vi "Enum Queue State Machine.vi"   [LabVIEW 2020, in "Enum Queue State Machine.lvlib"]
uses:
  Enum Queue State Machine.lvlib
  Enum Queue/Enqueue Enum (single).vi
  Toolbox/Controls State (array).vi
  Enum Queue/Enqueue Enum (array).vi
types:
  T1 = enum16{"User Event", "Initialize Core Data", "Data: Initialize", "Data: Cleanup", "UI: Initialize", "UI: Set Cursor State", "UI: Controls State", "UI: Front Panel State", "Macro: Initialize", "Macro: Exit", "Error Handler", "Exit"}
  T2 = enum32{"Invalid", "Standard", "Closed", "Hidden", "Minimized", "Maximized"}
  T3 = enum32{"invalid app kind", "Development System", "Run Time System", "Student Edition", "Embedded LabVIEW", "Evaluation", "Custom"}
  T4 = cluster{refnum<vi>[], "Disabled":enum8{"Enabled", "Disabled", "Disabled and Grayed Out"}}
  T5 = cluster{"Core":cluster{"Current VI Reference":refnum<vi>, "Close Panel on Exit?":bool}, "Data":bool}
  T6 = cluster{"Current VI Reference":refnum<vi>, "Close Panel on Exit?":bool}
  T7 = enum8{"Enabled", "Disabled", "Disabled and Grayed Out"}
  T8 = enum16{"User Event", "Initialize Core Data", "Data: Initialize", "Data: Cleanup", "UI: Initialize", "UI: Set Cursor State", "UI: Controls State", "UI: Front Panel State", "Macro: Initialize", "Macro: Exit", "Error Handler", "Exit"}[]
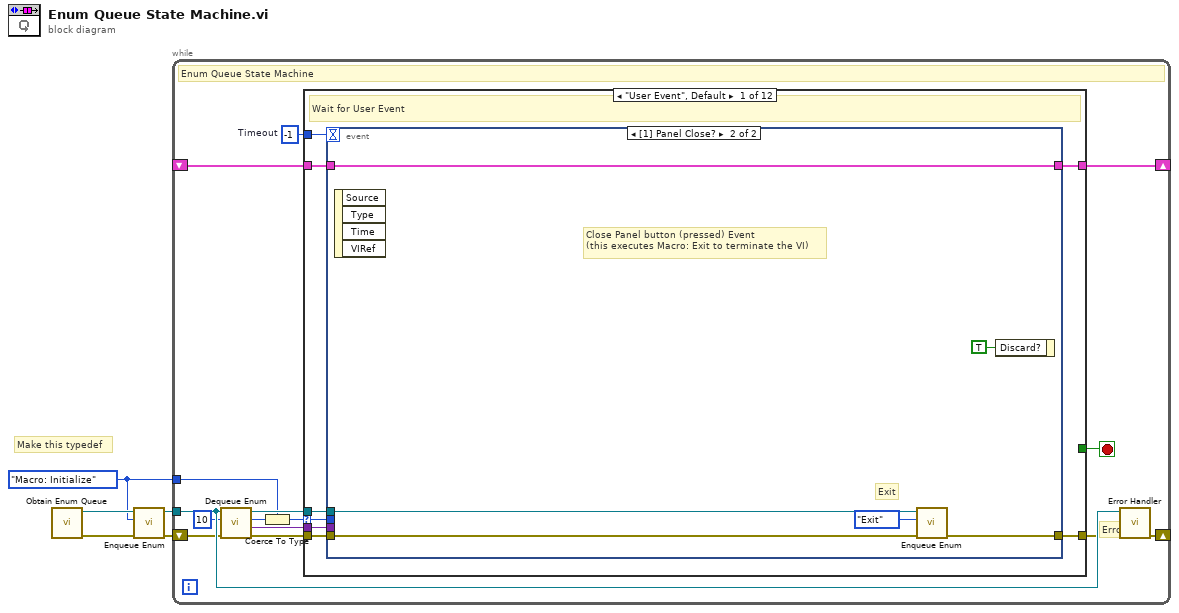
[diagram p0: block diagram]
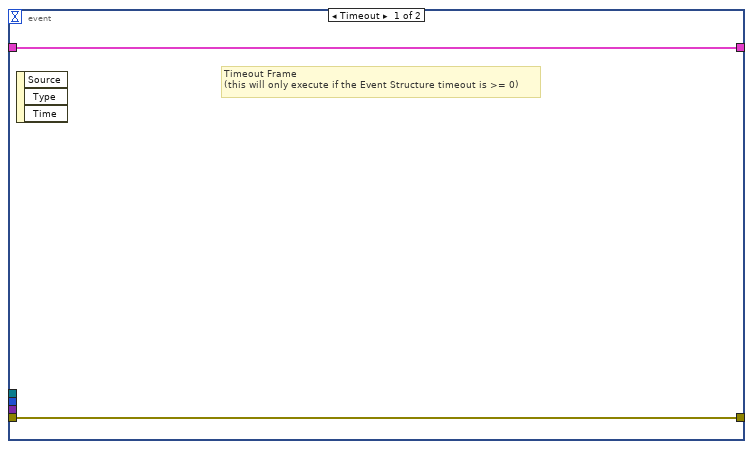
[diagram p2: hidden frame]
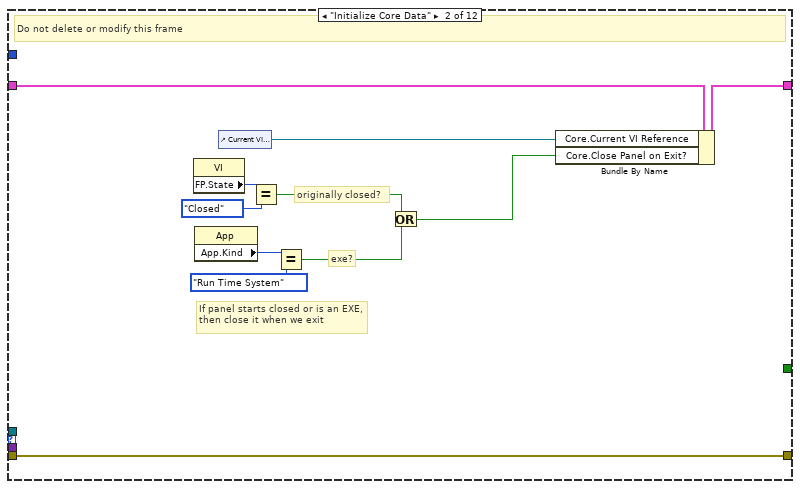
[diagram p3: hidden frame]
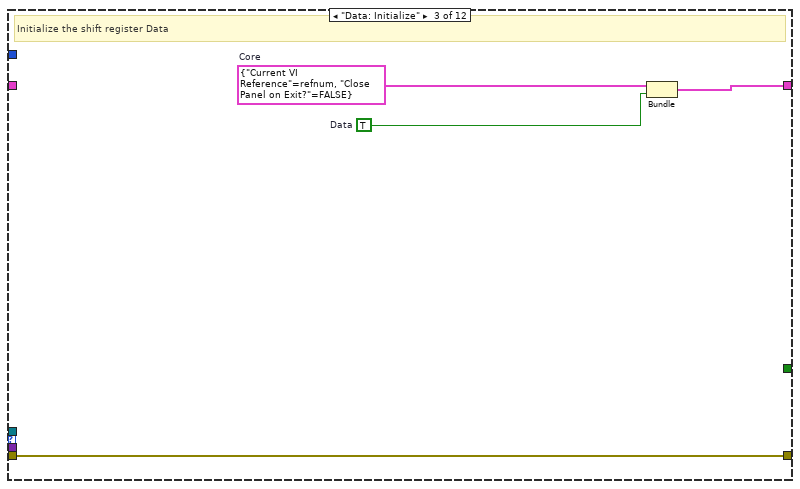
[diagram p4: hidden frame]
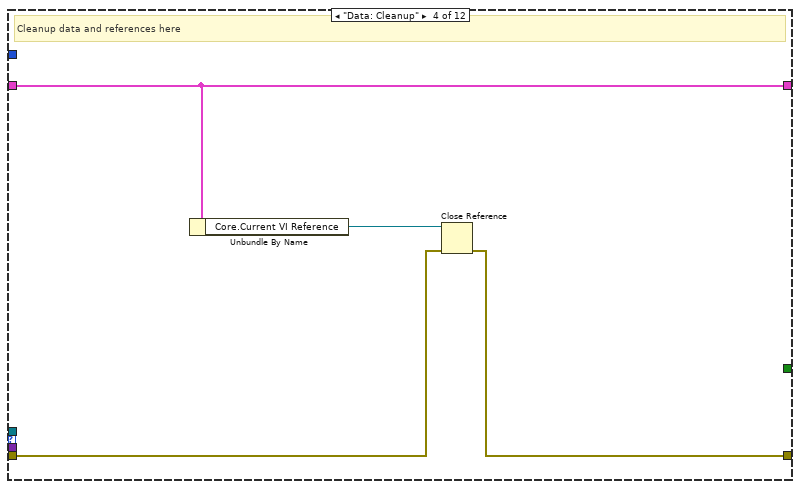
[diagram p5: hidden frame]
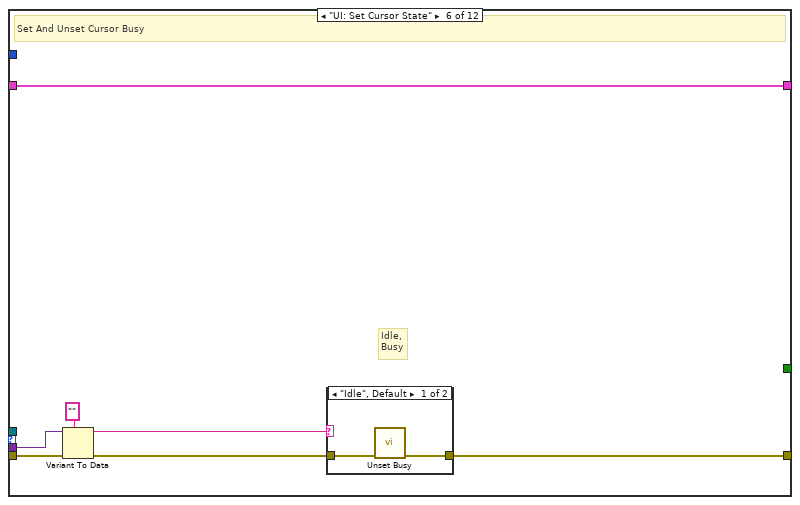
[diagram p7: hidden frame]
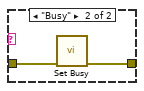
[diagram p8: hidden frame]
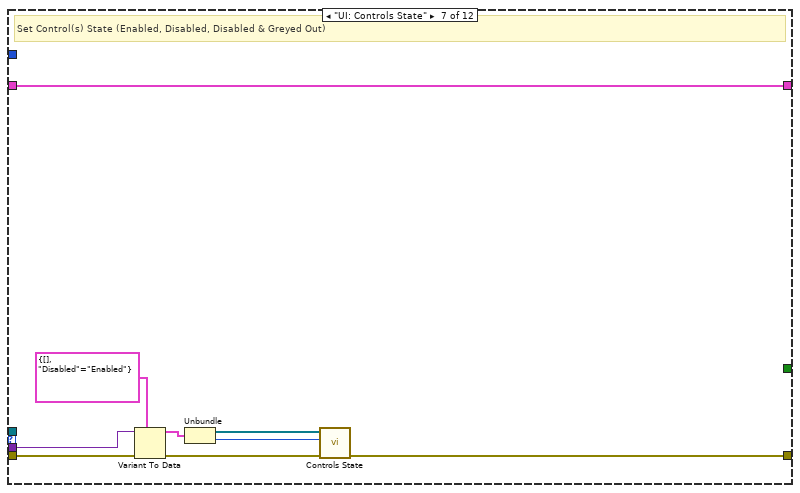
[diagram p9: hidden frame]
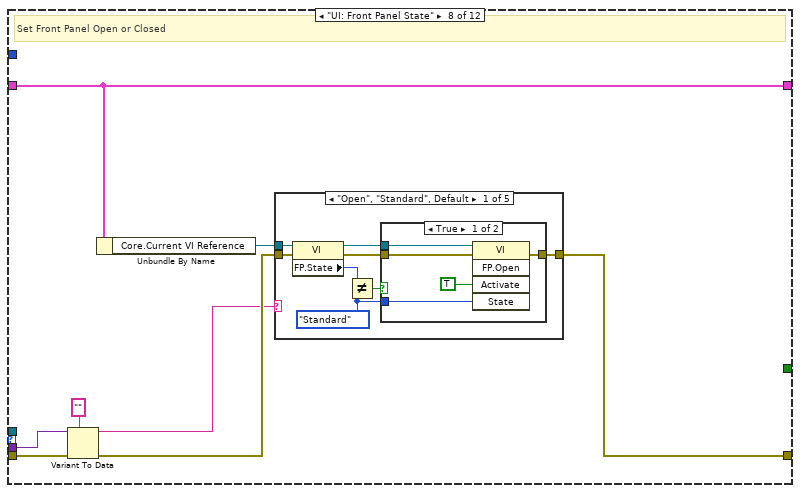
[diagram p10: hidden frame]
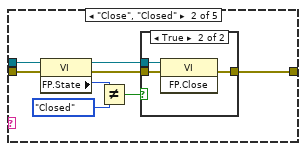
[diagram p12: hidden frame]
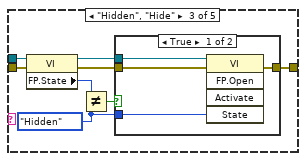
[diagram p14: hidden frame]
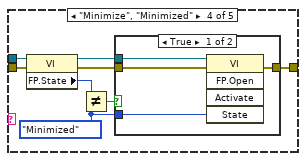
[diagram p16: hidden frame]
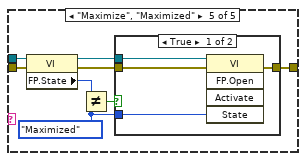
[diagram p18: hidden frame]
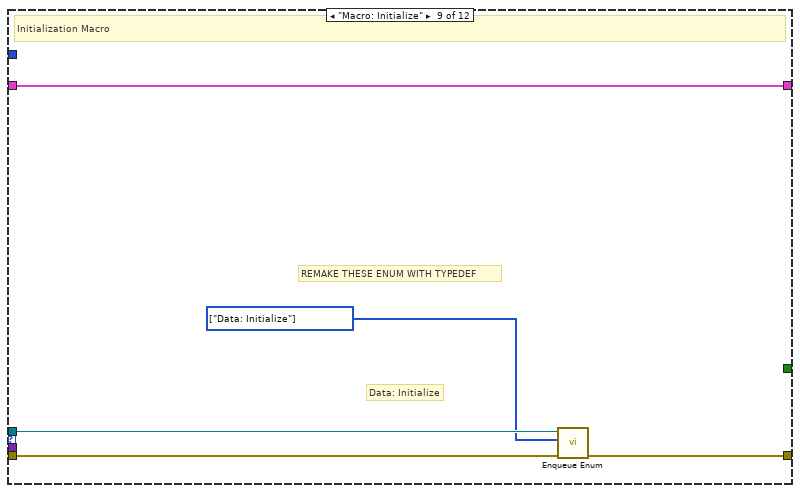
[diagram p20: hidden frame]
diagram:
  w1 = T1."Macro: Initialize"
  # "Make this typedef"
  n1 = call "Obtain Enum Queue.vi"() -> ("error out"=w2:errorcluster, "Queue Out"=w5:refnum<queue>)  [unwired: 10 in]
  n2 = call-poly "Enqueue Enum.vi"("error in"=w2, "State"=w1, "Queue In"=w5) -> ("error out"=w3:errorcluster, "Queue Out"=w4:refnum<queue>)  [unwired: 7 in]
  n3 = while {
    tunnel: w4 -> [w20]
    shift-right: [w6] -> _
    shift-left: w3 -> [w19]
    tunnel: w1 -> [w13]
    shift-right: [w11] -> _
    shift-left: _ -> [w12]
    stop <- w9 stop-if-true
    w10 = -1  # Timeout
    # "Error"
    # "Enum Queue State Machine"
    n4 = call "Dequeue Enum.vi"("error in"=w19, "Timeout ms (-1)"=10, "Queue In"=w20) -> ("error out"=w18:errorcluster, "Data"=w16:variant, "State"=w15:i32, "Queue Out"=w17:refnum<queue>)  [unwired: 5 in]
    n5 = Coerce To Type(0:w15, 1:w13) -> (2:w14:T1)
    n6 = case shown="\"User Event\", Default" w14 {
      selector: w14 -> [w21 _ _ _ _ _ _ _ _ _ _ _]
      tunnel: w18 -> [w28 w37 w51 w55 w57 w62 w76 w82 w154 w160 w175 w183]
      tunnel: w17 -> [w23 _ _ _ _ _ _ _ w152 w157 w174 w181]
      tunnel: w16 -> [w22 _ _ _ _ w60 w75 w80 _ _ _ _]
      tunnel: [w27 w37 w51 w54 w57 w63 w71 w84 w153 w163 w172 w182] -> w7
      tunnel: w12 -> [w25 w47 _ w53 w56 w64 w77 w83 w155 w161 w176 w185]
      tunnel: [w24 w46 w50 w53 w56 w64 w77 w83 w155 w161 w176 w185] -> w11
      tunnel: w10 -> [w26 _ _ _ _ _ _ _ _ _ _ _]
      tunnel: [_ _ _ _ _ _ _ _ _ _ _ TRUE] -> w9
      frame "User Event", Default {
        # "Wait for User Event"
        n7 = event shown="[1] Panel Close?" {
          selector: _ -> [_ _]
          dyn-events: _ -> [_ _]
          timeout: w26 -> [_ _]
          tunnel: w28 -> [w30 w34]
          tunnel: [w30 w33] -> w27
          tunnel: w25 -> [w29 w36]
          tunnel: [w29 w36] -> w24
          tunnel: w23 -> [_ w32]
          tunnel: w22 -> [_ _]
          tunnel: w21 -> [_ _]
          event Timeout {
            # "Timeout Frame\n(this will only execute if the Event Structure timeout is >= 0)"
            n8 = event-data() -> ()  [unwired: 1 in, 3 out]
          }
          event Panel Close? {
            # "Exit"
            # "Close Panel button (pressed) Event\n(this executes Macro: Exit to terminate the VI)"
            n9 = event-data() -> ()  [unwired: 1 in, 4 out]
            n10 = call-poly "Enqueue Enum.vi"("error in"=w34, "State"=T1."Exit", "Queue In"=w32) -> ("error out"=w33:errorcluster)  [unwired: 7 in, 1 out]
            n11 = event-data("Discard?"=TRUE) -> ()  [unwired: 1 in, 1 out]
          }
        }
      }
      frame "Initialize Core Data" {
        # "originally closed?"
        # "exe?"
        # "If panel starts closed or is an EXE, then close it when we exit"
        # "Do not delete or modify this frame"
        n12 = property class="VI"() -> ("FP.State"=w42:T2)  [unwired: 2 in, 2 out]
        n13 = property class="App"() -> ("App.Kind"=w45:T3)  [unwired: 2 in, 2 out]
        n14 = control-ref of="Current VI Reference"() -> (w39:refnum<vi>)
        n15 = Equal?(x=w42, y=T2."Closed" ("Front Panel Window:State")) -> (x = y?=w40:bool)
        n16 = Equal?(x=w45, y=T3."Run Time System" ("Application:Kind")) -> (x = y?=w43:bool)
        n17 = Or(x=w40, y=w43) -> (x .or. y?=w38:bool)
        n18 = Bundle By Name(cluster=w47, "Core.Current VI Reference"=w39, "Core.Close Panel on Exit?"=w38) -> (w46:T5)
      }
      frame "Data: Initialize" {
        w48 = TRUE  # Data
        w49 = T6 {"Current VI Reference"=refnum, "Close Panel on Exit?"=FALSE}  # Core
        # "Initialize the shift register Data"
        n19 = Bundle("Core"=w49, "Data"=w48) -> (w50:T5)  [unwired: 1 in]
      }
      frame "Data: Cleanup" {
        # "Cleanup data and references here"
        n20 = Unbundle By Name(w53) -> ("Core.Current VI Reference"=w52:refnum<vi>)
        n21 = Close Reference(reference=w52, error in (no error)=w55) -> (error out=w54:errorcluster)
      }
      frame "UI: Initialize" {
        # "Initialize the User Interface Here"
      }
      frame "UI: Set Cursor State" {
        # "Idle,\nBusy"
        # "Set And Unset Cursor Busy"
        n22 = Variant To Data(error in=w62, type="", Variant=w60) -> (data=w58:string, error out=w61:errorcluster)
        n23 = case shown="\"Idle\", Default" w58 {
          tunnel: w61 -> [w66 w68]
          tunnel: [w65 w67] -> w63
          frame "Idle", Default {
            n24 = call <vilib>:"Unset Busy.vi"("error in (no error)"=w66) -> ("error out"=w65:errorcluster)  [unwired: 10 in]
          }
          frame "Busy" {
            n25 = call <vilib>:"Set Busy.vi"("error in (no error)"=w68) -> ("error out"=w67:errorcluster)  [unwired: 9 in, 1 out]
          }
        }
      }
      frame "UI: Controls State" {
        # "Set Control(s) State (Enabled, Disabled, Disabled & Greyed Out)"
        n26 = Variant To Data(error in=w76, type=T4 {[], "Disabled"=enum."Enabled"}, Variant=w75) -> (data=w73:T4, error out=w72:errorcluster)
        n27 = Unbundle(w73) -> (w69:refnum<vi>[], "Disabled"=w70:T7)
        n28 = call-poly "Controls State.vi"("error in"=w72, "Disabled"=w70, "Controls Refnum"=w69) -> ("error out"=w71:errorcluster)  [unwired: 8 in]
      }
      frame "UI: Front Panel State" {
        # "Set Front Panel Open or Closed"
        n29 = Variant To Data(error in=w82, type="", Variant=w80) -> (data=w78:string, error out=w81:errorcluster)
        n30 = Unbundle By Name(w83) -> ("Core.Current VI Reference"=w85:refnum<vi>)
        n31 = case shown="\"Open\", \"Standard\", Default" w78 {
          tunnel: w81 -> [w91 w106 w117 w130 w143]
          tunnel: [w93 w107 w119 w132 w145] -> w84
          tunnel: w85 -> [w92 w104 w118 w131 w144]
          frame "Open", "Standard", Default {
            w86 = T2."Standard" ("State")
            n32 = property class="VI"(reference=w92, error in=w91) -> (reference out=w89:refnum<vi>, error out=w90:errorcluster, "FP.State"=w88:T2)
            n33 = Not Equal?(x=w88, y=w86) -> (x != y?=w87:bool)
            n34 = case shown="True" w87 {
              tunnel: [w97 w99] -> w93
              tunnel: w90 -> [w96 w99]
              tunnel: w89 -> [w95 _]
              tunnel: w86 -> [w94 _]
              frame True {
                n35 = invoke class="VI" method="FP.Open"(reference=w95, error in=w96, "Activate"=TRUE, "State"=w94) -> (error out=w97:errorcluster)  [unwired: 1 in, 4 out]
              }
              frame False {
              }
            }
          }
          frame "Close", "Closed" {
            n36 = property class="VI"(reference=w104, error in=w106) -> (reference out=w103:refnum<vi>, error out=w105:errorcluster, "FP.State"=w101:T2)
            n37 = Not Equal?(x=w101, y=T2."Closed" ("Front Panel Window:State")) -> (x != y?=w100:bool)
            n38 = case shown="True" w100 {
              tunnel: [w108 w111] -> w107
              tunnel: w105 -> [w108 w110]
              tunnel: w103 -> [_ w109]
              frame False {
              }
              frame True {
                n39 = invoke class="VI" method="FP.Close"(reference=w109, error in=w110) -> (error out=w111:errorcluster)  [unwired: 1 in, 2 out]
              }
            }
          }
          frame "Hidden", "Hide" {
            w112 = T2."Hidden" ("State")
            n40 = property class="VI"(reference=w118, error in=w117) -> (reference out=w115:refnum<vi>, error out=w116:errorcluster, "FP.State"=w114:T2)
            n41 = Not Equal?(x=w114, y=w112) -> (x != y?=w113:bool)
            n42 = case shown="True" w113 {
              tunnel: [w123 w124] -> w119
              tunnel: w116 -> [w122 w124]
              tunnel: w115 -> [w121 _]
              tunnel: w112 -> [w120 _]
              frame True {
                n43 = invoke class="VI" method="FP.Open"(reference=w121, error in=w122, "State"=w120) -> (error out=w123:errorcluster)  [unwired: 2 in, 4 out]
              }
              frame False {
              }
            }
          }
          frame "Minimize", "Minimized" {
            w125 = T2."Minimized" ("State")
            n44 = property class="VI"(reference=w131, error in=w130) -> (reference out=w128:refnum<vi>, error out=w129:errorcluster, "FP.State"=w127:T2)
            n45 = Not Equal?(x=w127, y=w125) -> (x != y?=w126:bool)
            n46 = case shown="True" w126 {
              tunnel: [w136 w137] -> w132
              tunnel: w129 -> [w135 w137]
              tunnel: w128 -> [w134 _]
              tunnel: w125 -> [w133 _]
              frame True {
                n47 = invoke class="VI" method="FP.Open"(reference=w134, error in=w135, "State"=w133) -> (error out=w136:errorcluster)  [unwired: 2 in, 4 out]
              }
              frame False {
              }
            }
          }
          frame "Maximize", "Maximized" {
            w138 = T2."Maximized" ("State")
            n48 = property class="VI"(reference=w144, error in=w143) -> (reference out=w141:refnum<vi>, error out=w142:errorcluster, "FP.State"=w140:T2)
            n49 = Not Equal?(x=w140, y=w138) -> (x != y?=w139:bool)
            n50 = case shown="True" w139 {
              tunnel: [w149 w150] -> w145
              tunnel: w142 -> [w148 w150]
              tunnel: w141 -> [w147 _]
              tunnel: w138 -> [w146 _]
              frame True {
                n51 = invoke class="VI" method="FP.Open"(reference=w147, error in=w148, "State"=w146) -> (error out=w149:errorcluster)  [unwired: 2 in, 4 out]
              }
              frame False {
              }
            }
          }
        }
      }
      frame "Macro: Initialize" {
        w151 = T8 [enum."Data: Initialize"] items=["User Event", "Initialize Core Data", "Data: Initialize", "Data: Cleanup", "UI: Initialize", "UI: Set Cursor State", "UI: Controls State", "UI: Front Panel State", "Macro: Initialize", "Macro: Exit", "Error Handler", "Exit"]
        # "Data: Initialize"
        # "REMAKE THESE ENUM WITH TYPEDEF"
        # "Initialization Macro"
        n52 = call-poly "Enqueue Enum.vi"("error in"=w154, "States"=w151, "Queue In"=w152) -> ("error out"=w153:errorcluster)  [unwired: 7 in, 1 out]
      }
      frame "Macro: Exit" {
        w162 = T8 [enum."Data: Cleanup", enum."Exit"] items=["User Event", "Initialize Core Data", "Data: Initialize", "Data: Cleanup", "UI: Initialize", "UI: Set Cursor State", "UI: Controls State", "UI: Front Panel State", "Macro: Initialize", "Macro: Exit", "Error Handler", "Exit"]
        # "Data: Cleanup\nExit"
        # "REMAKE THESE ENUM WITH TYPEDEF"
        # "Exit Macro"
        n53 = Unbundle By Name(w161) -> ("Core.Close Panel on Exit?"=w156:bool)
        n54 = case shown="True" w156 {
          tunnel: w160 -> [w164 w171]
          tunnel: [w164 w170] -> w159
          tunnel: [w165 w169] -> w158
          tunnel: w157 -> [w165 w168]
          frame False {
          }
          frame True {
            # "UI: Front Panel State"
            n55 = call-poly "Enqueue Enum.vi"("error in"=w171, "Data"="Close", "State"=T1."UI: Front Panel State", "Queue In"=w168) -> ("error out"=w170:errorcluster, "Queue Out"=w169:refnum<queue>)  [unwired: 6 in]
          }
        }
        n56 = call-poly "Enqueue Enum.vi"("error in"=w159, "States"=w162, "Queue In"=w158) -> ("error out"=w163:errorcluster)  [unwired: 7 in, 1 out]
      }
      frame "Error Handler" {
        # "Error States"
        # "Clear error"
        # "Unhandled Error -- Display it"
        # "Hendle Any Error Here"
        n57 = call <vilib>:"General Error Handler.vi"("error in (no error)"=w175) -> ()  [unwired: 10 in, 5 out]
        n58 = disable-structure shown="Disabled" {
          disable-tunnel: w174 -> [w179 _]
          disable-tunnel: errorcluster {"status"=FALSE, "code"=0, "source"=""} ("error out") -> [w178 w180]
          disable-tunnel: [w177 w180] -> w172
          frame Disabled {
            n59 = call-poly "Enqueue Enum.vi"("error in"=w178, "Queue In"=w179) -> ("error out"=w177:errorcluster)  [unwired: 8 in, 1 out]
          }
          frame Enabled {
          }
        }
      }
      frame "Exit" {
        # "Hendle Any Error Here"
        n60 = Release Queue(queue=w181, error in (no error)=w183) -> (error out=w182:errorcluster)  [unwired: 1 in, 2 out]
      }
    }
    n61 = call "Error Handler.vi"("error in (no error)"=w7, "Queue In"=w20) -> ("dup error in"=w6:errorcluster)  [unwired: 8 in, 1 out]
  }
